vi "TW_WriteData.vi"(8 "number":dbl, 9 "value":string, 11 "Property":string) -> ()   [LabVIEW 2019]
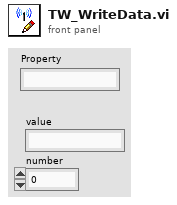
[diagram p1: front panel]
types:
  T1 = enum16{"GET", "PUT", "POST", "MultiPOST", "DELETE"}
  T2 = cluster{"Name":string, "BaseURL":string, "AppKey":string, "Headers":string[], "Timeout":i32}
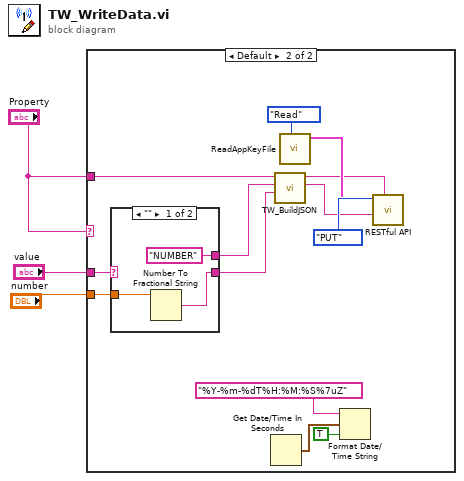
[diagram p0: block diagram]
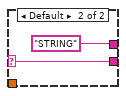
[diagram p3: hidden frame]
diagram:
  n1 = case shown="Default" "Property" {
    tunnel: "Property" -> [_ w10]
    tunnel: "value" -> [_ w6]
    tunnel: "number" -> [_ w4]
    frame "" {
    }
    frame Default {
      n2 = case shown="\"\"" w6 {
        selector: w6 -> [_ w20]
        tunnel: ["NUMBER" ("type") "STRING" ("type")] -> w7
        tunnel: [w18 w20] -> w5
        tunnel: w4 -> [w19 _]
        frame "" {
          n3 = Number To Fractional String(number=w19) -> (F-format string=w18:string)  [unwired: 3 in]
        }
        frame Default {
        }
      }
      n4 = Get Date/Time In Seconds() -> (seconds since 1Jan1904=w15:timestamp)
      n5 = call "TW_BuildJSON.vi"("Value"=w5, "type"=w7, "Thingworx"=w10) -> ("JSON"=w8:string, "URL"=w9:string)  [unwired: 7 in]
      n6 = call "ReadAppKeyFile.vi"("Task"=enum16{"Read", "Write"}."Read") -> ("Device Out"=w11:T2)  [unwired: 8 in, 2 out]
      n7 = Format Date/Time String(time format string (%c)="%Y-%m-%dT%H:%M:%S%7uZ", seconds (now)=w15, UTC format=TRUE) -> ()  [unwired: 1 out]
      n8 = call "RESTful API.vi"("Method"=T1."PUT", "url"=w9, "JSON"=w8, "Device In"=w11) -> ()  [unwired: 5 in, 3 out]
    }
  }
